vi "Game Board_Init.vi"(8 "error in (no error)":errorcluster, 9 "Board Size":T1={"X"=10, "Y"=20}, 10 "Board color":u32(colorbox)=13816530) -> (0 "error out":errorcluster, 3 "object out":refnum<class "Game Board.lvclass">)   [LabVIEW 2017, in "Game Board.lvclass"]
uses:
  Game Board.lvclass
  Controls/Coordinates.ctl
  Game Board.lvclass/Game Board.ctl
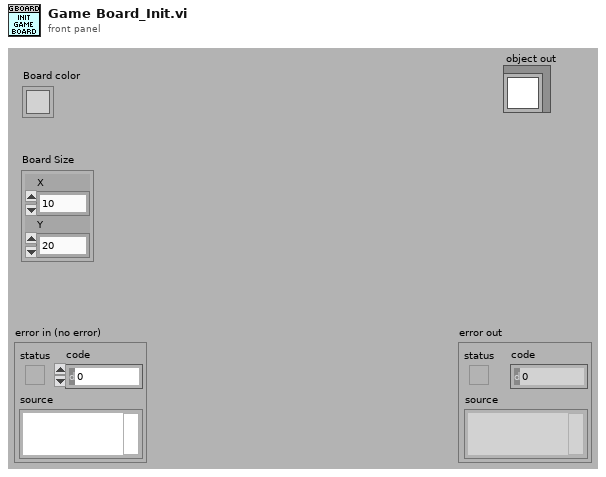
[diagram p1: front panel]
types:
  T1 = typedef "Coordinates.ctl" = cluster{"X":i32, "Y":i32}
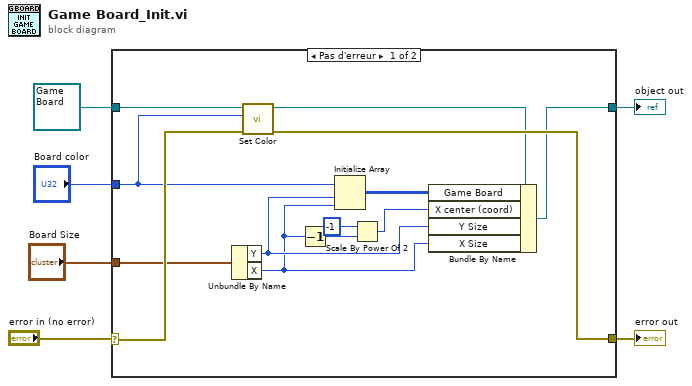
[diagram p0: block diagram]
diagram:
  n1 = case shown="Pas d'erreur" "error in (no error)" {
    selector: "error in (no error)" -> [w19 w20]
    tunnel: [w17 w21] -> w6
    tunnel: refnum<class "Game Board.lvclass"> refnum ("object in") -> [w16 w21]
    tunnel: [w18 w20] -> w3
    tunnel: "Board color" -> [w14 _]
    tunnel: "Board Size" -> [w12 _]
    frame No Error {
      n2 = Unbundle By Name(w12) -> ("Y"=w8:i32, "X"=w7:i32)
      n3 = call-dynamic "Set Color.vi"("error in (no error)"=w19, "Color"=w14, "object in"=w16) -> ("error out"=w18:errorcluster, "object out"=w15:refnum<class "Game Board.lvclass">)  [unwired: 7 in]
      n4 = Decrement(x=w7) -> (x-1=w10:i32)
      n5 = Initialize Array(w14, w8, w7) -> (w13:u32[][])
      n6 = Scale By Power Of 2(n=i16 -1, x=w10) -> (x*2^n=w11:i32)
      n7 = Bundle By Name(cluster=w15, "Game Board"=w13, "X center (coord)"=w11, "Y Size"=w8, "X Size"=w7) -> (w17:refnum<class "Game Board.lvclass">)
    }
    frame Error {
    }
  }
  "object out" <- w6
  "error out" <- w3
